vi "HW_Server_memory.vi"(6 "Modules Aliases List In":string[][](array[string]), 7 "Operation":T1=enum."WRITE", 8 "error in":errorcluster, 9 "Modules In":string[][](array[string]), 10 "Chassis Alias List In":string[](array[string]), 11 "Chassis List In":string[](array[string])) -> (0 "error out":errorcluster, 2 "All Variables Out":string[](array[string]), 3 "Data Ref Out":variant[](array[variant]))   [LabVIEW 2011]
doc: "This VI will store the config data."
uses:
  Controls/Read - Write.ctl
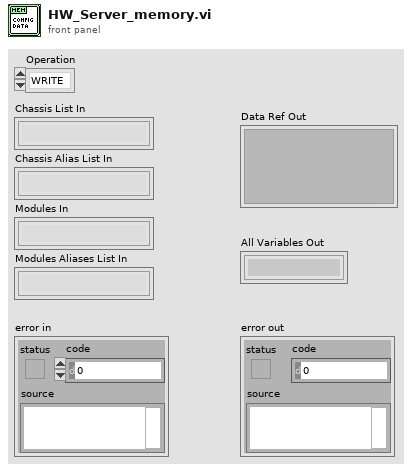
[diagram p1: front panel]
types:
  T1 = typedef "Read - Write.ctl" = enum16{"READ", "WRITE"}
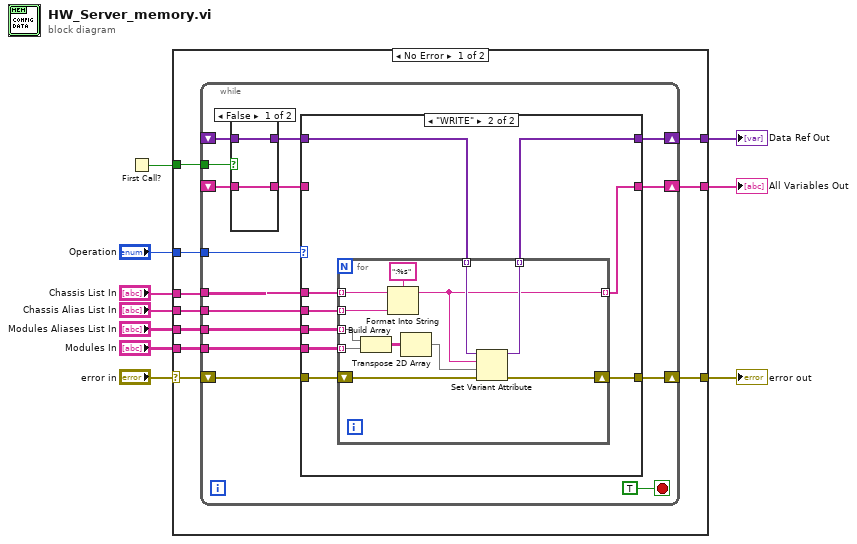
[diagram p0: block diagram]
diagram:
  n1 = First Call?() -> (First Call?: T/F=w1:bool)
  n2 = case shown="No Error" "error in" {
    selector: "error in" -> [w12 w62]
    tunnel: "Modules Aliases List In" -> [w20 _]
    tunnel: "Modules In" -> [w19 _]
    tunnel: "Chassis List In" -> [w18 _]
    tunnel: "Chassis Alias List In" -> [w17 _]
    tunnel: "Operation" -> [w16 _]
    tunnel: [w15 w62] -> w5
    tunnel: [w14 _] -> w4
    tunnel: [w13 _] -> w3
    tunnel: w1 -> [w11 _]
    frame No Error {
      n3 = while {
        tunnel: w18 -> [w31]
        tunnel: w17 -> [w32]
        tunnel: w20 -> [w30]
        tunnel: w19 -> [w29]
        shift-right: [w34] -> w15
        shift-left: w12 -> [w35]
        shift-right: [w33] -> w13
        shift-left: _ -> [w23]
        shift-right: [w28] -> w14
        shift-left: _ -> [w25]
        tunnel: w16 -> [w27]
        tunnel: w11 -> [w21]
        stop <- TRUE stop-if-true
        n4 = case shown="False" w21 {
          tunnel: w25 -> [w37 _]
          tunnel: [w37 _] -> w24
          tunnel: w23 -> [w36 _]
          tunnel: [w36 _] -> w22
          frame False {
          }
          frame True {
          }
        }
        n5 = case shown="\"WRITE\"" w27 {
          tunnel: w35 -> [w40 w49]
          tunnel: [w40 w48] -> w34
          tunnel: [w38 w47] -> w33
          tunnel: w22 -> [w38 w46]
          tunnel: w32 -> [_ w45]
          tunnel: w31 -> [_ w44]
          tunnel: w30 -> [_ w43]
          tunnel: w29 -> [_ w42]
          tunnel: [w39 w41] -> w28
          tunnel: w24 -> [w39 _]
          frame "READ" {
          }
          frame "WRITE" {
            n6 = for {
              tunnel: [w60] -> w47 mode=indexing
              tunnel: w46 -> [w59] mode=indexing
              tunnel: w45 -> [w56] mode=indexing
              tunnel: w44 -> [w57] mode=indexing
              tunnel: w43 -> [w54] mode=indexing
              tunnel: w42 -> [w53] mode=indexing
              shift-right: [w55] -> w48
              shift-left: w49 -> [w61]
              tunnel: [w52] -> w41 mode=indexing
              n7 = Build Array(w54, w53) -> (w51:string[][])
              n8 = Format Into String(format string=":%s", initial string=w57, w56) -> (resulting string=w52:string)  [unwired: 1 in, 1 out]
              n9 = Transpose 2D Array(2D array=w51) -> (transposed array=w50:string[][])
              n10 = Set Variant Attribute(Variant=w59, name=w52, value=w50, error in=w61) -> (Variant out=w60:variant, error out=w55:errorcluster)  [unwired: 1 out]
            }
          }
        }
      }
    }
    frame Error {
    }
  }
  "error out" <- w5
  "All Variables Out" <- w4
  "Data Ref Out" <- w3
